vi "Tower Light.vi"(9 "String":string, 10 "Type":u8, 11 "Index":u8) -> (3 "Succeed?":bool, 4 "error out":errorcluster)   [LabVIEW 2020, in "FBN_LATM.lvlib"]
uses:
  FBN_LATM.lvlib
panel:
  out "return type":u8
  out "appended path":path
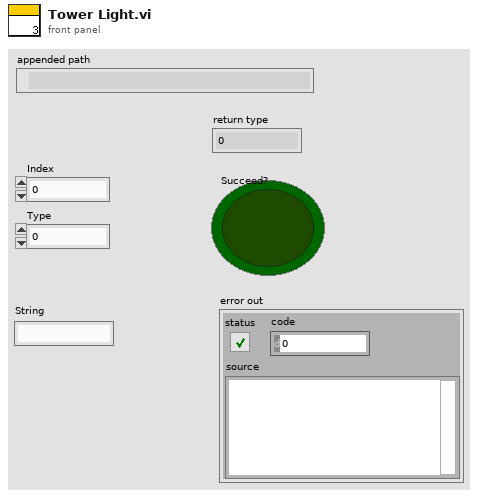
[diagram p1: front panel]
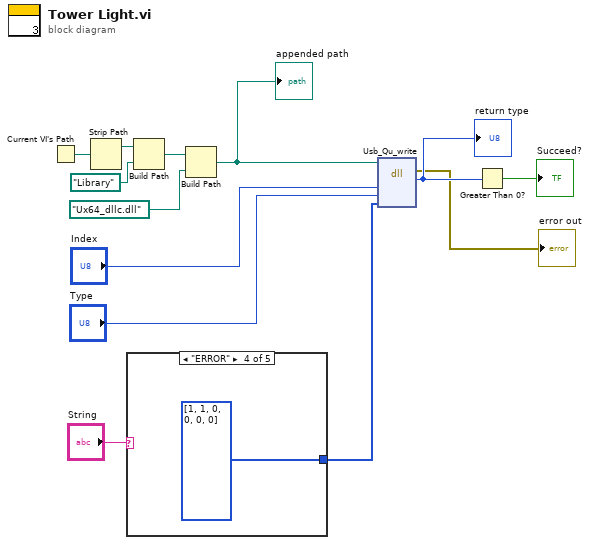
[diagram p0: block diagram]
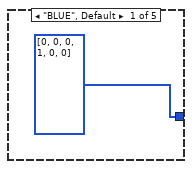
[diagram p2: hidden frame]
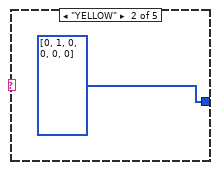
[diagram p3: hidden frame]
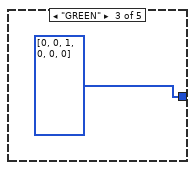
[diagram p4: hidden frame]
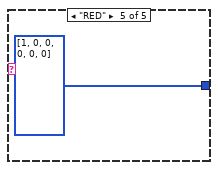
[diagram p5: hidden frame]
diagram:
  n1 = Current VI's Path() -> (path=w13:path)
  n2 = Strip Path(path=w13) -> (stripped path=w12:path)  [unwired: 1 out]
  n3 = case shown="\"ERROR\"" "String" {
    tunnel: [u8[] [0, 0, 0, 1, 0, 0] ("Data 2") u8[] [0, 1, 0, 0, 0, 0] ("Data 2") u8[] [0, 0, 1, 0, 0, 0] ("Data 2") u8[] [1, 1, 0, 0, 0, 0] ("Data 2") u8[] [1, 0, 0, 0, 0, 0] ("Data 2")] -> w1
    frame "BLUE", Default {
    }
    frame "YELLOW" {
    }
    frame "GREEN" {
    }
    frame "ERROR" {
    }
    frame "RED" {
    }
  }
  n4 = Build Path(base path=w12, name or relative path=path "Library") -> (appended path=w10:path)
  n5 = Build Path(base path=w10, name or relative path=path "Ux64_dllc.dll") -> (appended path=w8:path)
  "appended path" <- w8
  n6 = dll-call lib="C:/Project/031210-COMMON CORE/Software/Sources/Drivers/Signalworks USB56/Ux64_dllc.dll" fn="Usb_Qu_write"(path in=w8, "Index"="Index", "Type"="Type", "Data"=w1) -> (error out=→"error out":errorcluster, "return type"=w7:u8)  [unwired: 5 in, 1 out]
  "return type" <- w7
  n7 = Greater Than 0?(x=w7) -> (x > 0?=→"Succeed?":bool)
